vi "Initialize Instrument.vi"(8 "error in (no error)":errorcluster, 10 "Reset":bool, 11 "Agilent 428x in":refnum<class "Agilent 428x.lvclass">) -> (0 "error out":errorcluster, 3 "Agilent 428x out":refnum<class "Agilent 428x.lvclass">)   [LabVIEW 2020, in "Agilent 428x.lvclass"]
uses:
  Agilent 428x.lvclass
  C:/Sandbox/Git_Sandbox/WiSpry Test Framework source code (LV20)/WiSpry Test Framework/Instruments/Instrument.lvclass
  Instrument.lvclass/Instrument.ctl
  Instrument.lvclass
  <instrlib>/Agilent 428X Series/Agilent 428X Series.lvlib
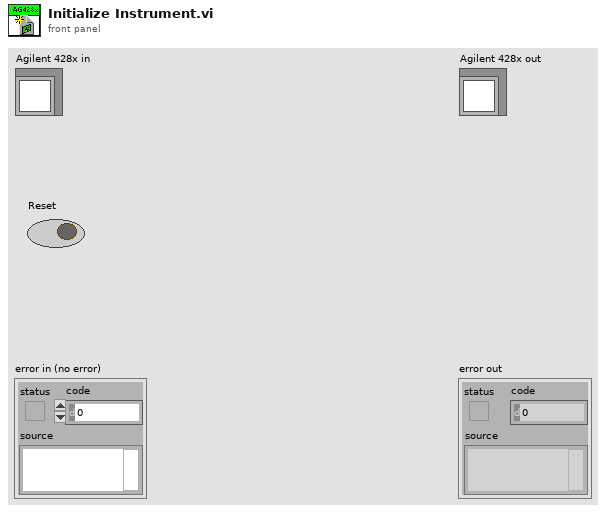
[diagram p1: front panel]
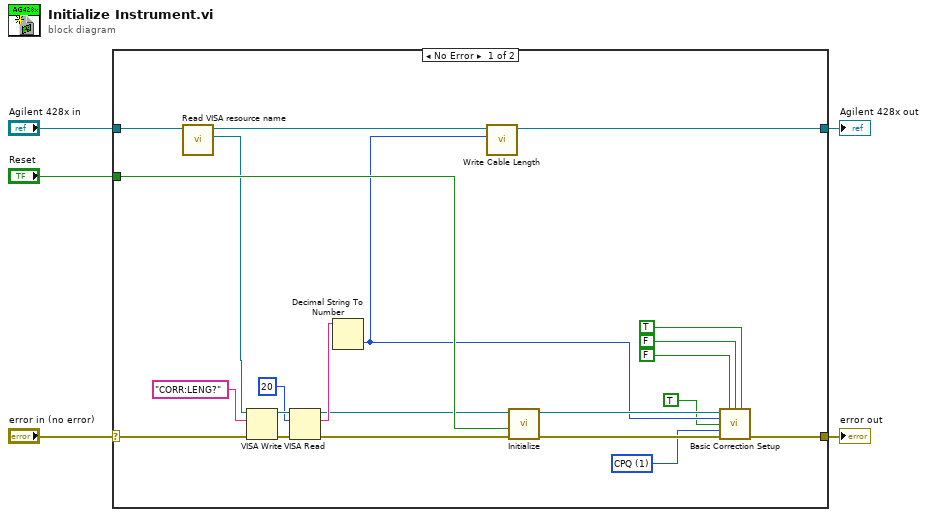
[diagram p0: block diagram]
diagram:
  n1 = case shown="No Error" "error in (no error)" {
    selector: "error in (no error)" -> [w15 w29]
    tunnel: [w25 w29] -> w4
    tunnel: [w12 w28] -> w3
    tunnel: "Agilent 428x in" -> [w27 w28]
    tunnel: "Reset" -> [w26 _]
    frame No Error {
      w8 = u32 1 items=["CPD", "CPQ", "CPG", "CPRP", "CSD", "CSQ", "CSRS", "LPQ", "LPD", "LPG", "LPRP", "LSD", "LSQ", "LSRS", "RX", "ZTD", "ZTR", "GB", "YTD", "YTR"] ("Load Type (0: CPD)")
      n2 = call "Read VISA resource name.vi"("Instrument in"=w27) -> ("VISA resource name"=w17:refnum<visa-resource-name>, "Instrument out"=w13:refnum<class "Agilent 428x.lvclass">)  [unwired: 9 in]
      n3 = VISA Write(VISA resource name=w17, write buffer="CORR:LENG?", error in (no error)=w15) -> (VISA resource name out=w22:refnum<visa-resource-name>, error out=w21:errorcluster)  [unwired: 1 out]
      n4 = VISA Read(VISA resource name=w22, byte count=u32 20, error in (no error)=w21) -> (VISA resource name out=w16:refnum<visa-resource-name>, read buffer=w18:string, error out=w14:errorcluster)  [unwired: 1 out]
      n5 = Decimal String To Number(string=w18) -> (number=w11:i32)  [unwired: 2 in, 1 out]
      n6 = call-dynamic "Write Cable Length.vi"("Cable Length (0: 0 m)"=w11, "Agilent 428x in"=w13) -> ("Agilent 428x out"=w12:refnum<class "Agilent 428x.lvclass">)  [unwired: 8 in, 1 out]
      n7 = call <instrlib>:"Initialize.vi"("error in (no error)"=w14, "Reset (T: Reset)"=w26, "VISA resource name"=w16) -> ("error out"=w24:errorcluster, "VISA resource name out"=w23:refnum<visa-resource-name>)  [unwired: 7 in]
      n8 = call <instrlib>:"Basic Correction Setup.vi"("VISA resource name"=w23, "Load Corr  (F: Off)"=FALSE ("Short Corr (T: On)"), "Short Corr (T: On)"=FALSE, "Open Corr  (F: Off)"=TRUE, "Cable Length (0: 4 m)"=w11, "Corr Method (T: Single)"=TRUE, "Load Type (0: CPD)"=w8, "error in (no error)"=w24) -> ("error out"=w25:errorcluster)  [unwired: 5 in, 2 out]
    }
    frame Error {
    }
  }
  "error out" <- w4
  "Agilent 428x out" <- w3
